vi "Calibrate.vi"(8 "error in (no error)":errorcluster, 10 "Perform Auto Calibration":bool, 11 "LockinDAQ in":refnum<class "LockinDAQ.lvclass">) -> (0 "error out":errorcluster, 2 "Cal Info":T1[](array[typedef]), 3 "LockinDAQ out":refnum<class "LockinDAQ.lvclass">)   [LabVIEW 2016, in "LockinDAQ.lvclass"]
uses:
  LockinDAQ.lvclass
  Typedefs/Cal Info - Cluster.ctl
  LockinDAQ.lvclass/LockinDAQ.ctl
  <vilib>/addons/WireFlow/_WF_ProgressBar.llb/WindowBehavior.ctl
  <userlib>/_OpenG.lib/array/array.llb/Remove Duplicates from 1D Array (String)__ogtk.vi
  <vilib>/addons/WireFlow/_WF_ProgressBar.llb/ProgressBar_WireFlow.lvclass
  <resource>/objmgr/daqmx.rc
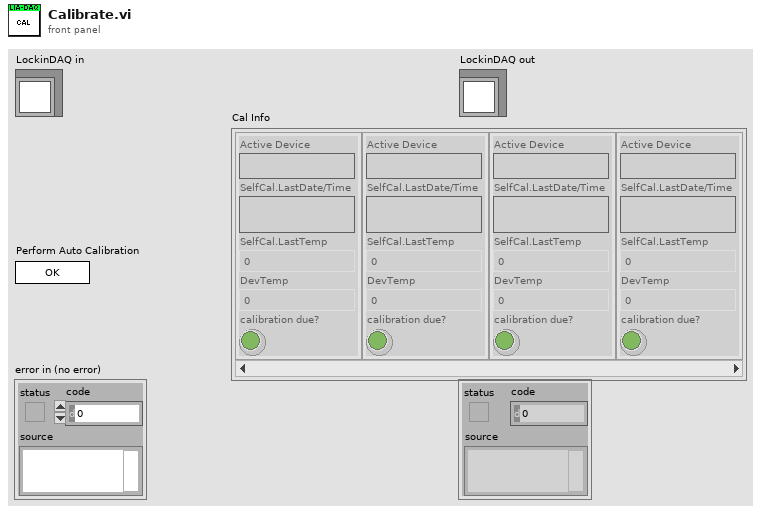
[diagram p1: front panel]
types:
  T1 = typedef "Cal Info - Cluster.ctl" = cluster{"Active Device":string, "SelfCal.LastDate/Time":string, "SelfCal.LastTemp":dbl, "DevTemp":dbl, "calibration due?":bool}
  T2 = typedef "ProgressBar_WireFlow.lvclass/WindowBehavior.ctl" = enum16{"No change", "Modal", "Floating"}
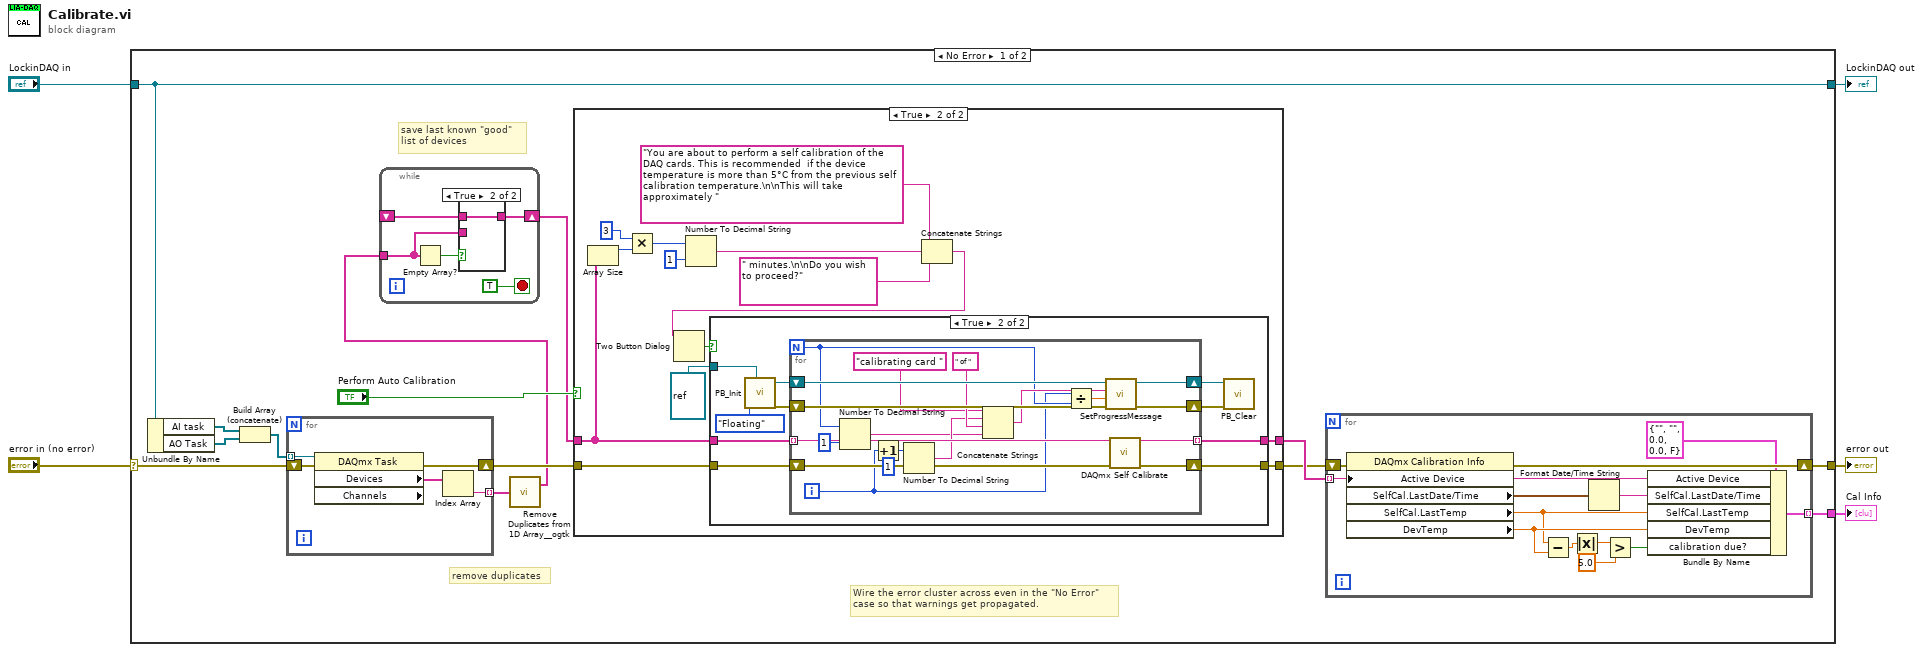
[diagram p0: block diagram]
diagram:
  n1 = case shown="No Error" "error in (no error)" {
    selector: "error in (no error)" -> [w8 w92]
    tunnel: [w7 w92] -> w4
    tunnel: [w12 w91] -> w2
    tunnel: "LockinDAQ in" -> [w12 w91]
    tunnel: [w9 _] -> w1
    frame No Error {
      # "save last known \"good\"\nlist of devices"
      # "remove duplicates"
      # "Wire the error cluster across even in the \"No Error\"\ncase so that warnings get propagated."
      n2 = Unbundle By Name(w12) -> ("AI task"=w11:refnum<k21>[], "AO Task"=w10:refnum<k21>[])
      n3 = Build Array (concatenate)(w11, w10) -> (w6:refnum<k21>[])
      n4 = for {
        tunnel: [w35] -> w19 mode=indexing
        shift-right: [w36] -> w18
        shift-left: w8 -> [w37]
        tunnel: w6 -> [w33] mode=indexing
        n5 = property class="DAQmx Task" props=["Devices", "Channels"](reference=w33, error in=w37) -> (error out=w36:errorcluster, "Devices"=w34:tag[])  [unwired: 2 out]
        n6 = Index Array(array=w34) -> (element=w35:tag)  [unwired: 1 in]
      }
      n7 = call-poly <userlib>:"Remove Duplicates from 1D Array__ogtk.vi"("Input Array"=w19) -> ("Output Array"=w14:string[])  [unwired: 1 out]
      n8 = while {
        shift-right: [w40] -> w13
        shift-left: _ -> [w38]
        tunnel: w14 -> [w39]
        stop <- TRUE stop-if-true
        n9 = Empty Array?(array=w39) -> (empty?=w41:bool)
        n10 = case shown="True" w41 {
          tunnel: [w43 w44] -> w40
          tunnel: w39 -> [w43 _]
          tunnel: w38 -> [_ w44]
          frame False {
          }
          frame True {
          }
        }
      }
      n11 = case shown="True" "Perform Auto Calibration" {
        tunnel: w18 -> [w46 w60]
        tunnel: [w46 w59] -> w16
        tunnel: w13 -> [w45 w57]
        tunnel: [w45 w58] -> w17
        frame False {
        }
        frame True {
          n12 = Array Size(array=w57) -> (size(s)=w56:i32)
          n13 = Multiply(x=3, y=w56) -> (x*y=w48:i32)
          n14 = Number To Decimal String(number=w48, width (-)=i16 1) -> (decimal integer string=w49:string)
          n15 = Concatenate Strings("You are about to perform a self calibration of the DAQ cards. This is recommended  if the device temperature is more than 5°C from the previous self calibration temperature.\n\nThis will take approximately " ("message"), w49, " minutes.\n\nDo you wish to proceed?") -> (w50:string)
          n16 = Two Button Dialog(message=w50) -> (T button?=w51:bool)  [unwired: 2 in]
          n17 = case shown="True" w51 {
            tunnel: w60 -> [w62 w72]
            tunnel: [w62 w71] -> w59
            tunnel: [w61 w70] -> w58
            tunnel: w57 -> [w61 w69]
            tunnel: refnum<vi> refnum ("Progress VI") -> [_ w64]
            frame False {
            }
            frame True {
              n18 = call <vilib>:"PB_Init.vi"("Progress VI"=w64, "Window behavior (No change)"=WindowBehavior."Floating") -> ("error out"=w65:errorcluster, "WF-ProgressBar out"=w66:refnum<class "ProgressBar_WireFlow.lvclass">)  [unwired: 8 in]
              n19 = for {
                N -> [w79]
                shift-right: [w89] -> w71
                shift-left: w72 -> [w90]
                tunnel: w69 -> [w88] mode=indexing
                tunnel: [w88] -> w70 mode=indexing
                shift-right: [w85] -> w68
                shift-left: w66 -> [w86]
                shift-right: [w84] -> w67
                shift-left: w65 -> [w87]
                i -> [w74]
                n20 = Number To Decimal String(number=w79, width (-)=i16 1) -> (decimal integer string=w75:string)
                n21 = Increment(x=w74) -> (x+1=w73:i32)
                n22 = Number To Decimal String(number=w73, width (-)=i16 1) -> (decimal integer string=w77:string)
                n23 = Concatenate Strings("calibrating card ", w77, " of ", w75) -> (w80:string)
                n24 = Divide(x=w74, y=w79) -> (x/y=w81:dbl)
                n25 = call-dynamic "SetProgressMessage.vi"("error in (no error)"=w87, "Progress value (NaN no update)"=w81, "Message"=w80, "WF-ProgressBar in"=w86) -> ("error out"=w84:errorcluster, "WF-ProgressBar out"=w85:refnum<class "ProgressBar_WireFlow.lvclass">)  [unwired: 5 in, 1 out]
                n26 = call <vilib>:"DAQmx Self Calibrate.vi"("device in"=w88, "error in"=w90) -> ("error out"=w89:errorcluster)  [unwired: 13 in]
              }
              n27 = call-dynamic "PB_Clear.vi"("error in (no error)"=w67, "WF-ProgressBar in"=w68) -> ()  [unwired: 8 in, 2 out]
            }
          }
        }
      }
      n28 = for {
        tunnel: [w31] -> w9 mode=indexing
        shift-right: [w32] -> w7
        shift-left: w16 -> [w30]
        tunnel: w17 -> [w20] mode=indexing
        n29 = property class="DAQmx Calibration Info"(error in=w30, "Active Device"=w20) -> (error out=w32:errorcluster, "SelfCal.LastDate/Time"=w26:timestamp, "SelfCal.LastTemp"=w21:dbl, "DevTemp"=w22:dbl)  [unwired: 1 in, 1 out]
        n30 = Subtract(x=w21, y=w22) -> (x-y=w24:dbl)
        n31 = Absolute Value(x=w24) -> (abs(x)=w29:dbl)
        n32 = Format Date/Time String(seconds (now)=w26) -> (date/time string=w25:string)  [unwired: 2 in]
        n33 = Greater?(x=w29, y=5.0) -> (0:w23:bool)
        n34 = Bundle By Name(cluster=T1 {"Active Device"="", "SelfCal.LastDate/Time"="", "SelfCal.LastTemp"=0.0, "DevTemp"=0.0, "calibration due?"=FALSE} ("System Cluster"), "Active Device"=w20, "SelfCal.LastDate/Time"=w25, "SelfCal.LastTemp"=w21, "DevTemp"=w22, "calibration due?"=w23) -> (w31:T1)
      }
    }
    frame Error {
    }
  }
  "error out" <- w4
  "LockinDAQ out" <- w2
  "Cal Info" <- w1
